vi "Clear_TemporaryFiles.vi"() -> ()   [LabVIEW 2018]
panel:
  out "text":string
  in  "EventCodes_U64Arr in":u64[](array[numeric])
  out "data":u64[](array[numeric])
  out "All Files in Dir":path[](array[path])
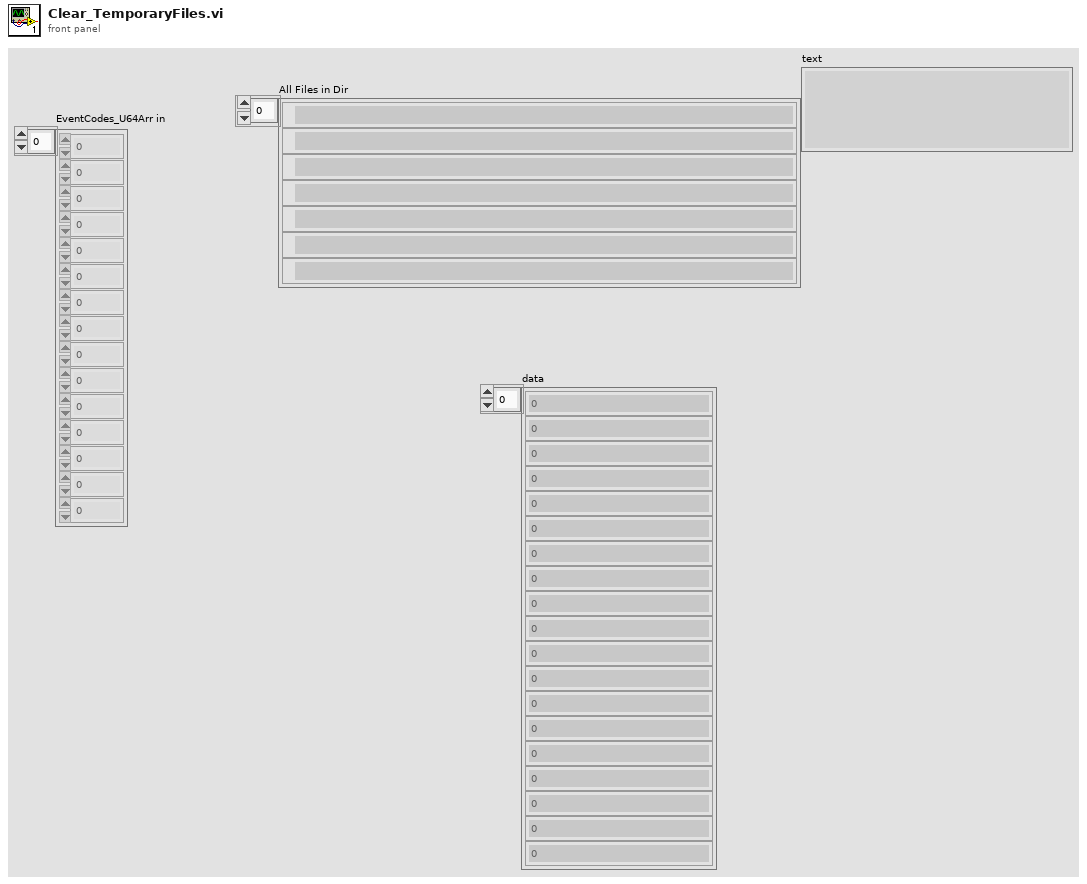
[diagram p1: front panel]
types:
  T1 = enum16{"open", "replace", "create", "open or create", "replace or create", "replace or create with confirmation"}
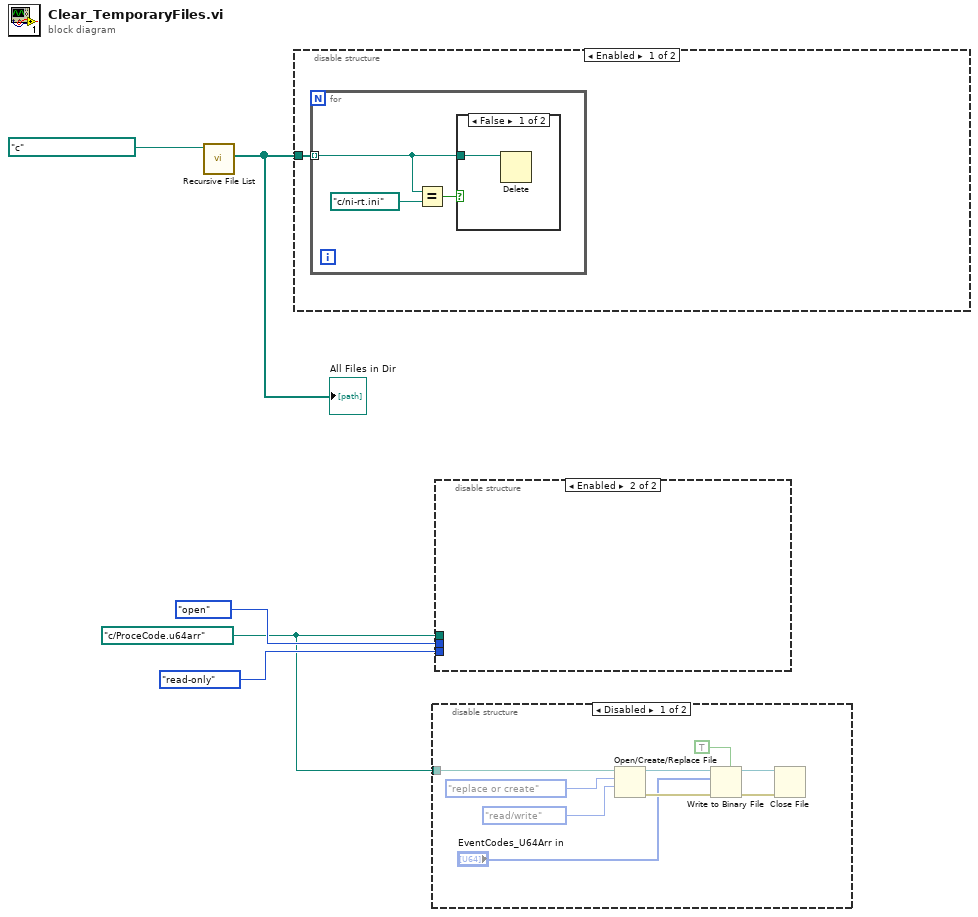
[diagram p0: block diagram]
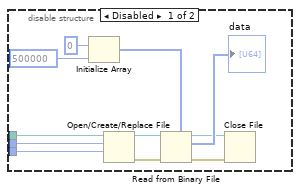
[diagram p3: hidden frame]
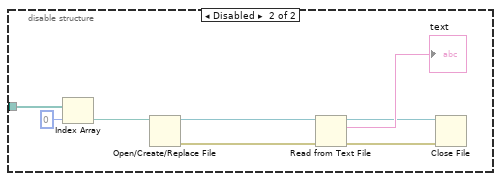
[diagram p5: hidden frame]
diagram:
  w2 = path "c:/ProceCode.u64arr" ("file path (use dialog)")
  n1 = call <vilib>:"Recursive File List.vi"("Folder Path"=path "c:/" ("file path (use dialog)")) -> ("All Files in Dir"=w1:path[])  [unwired: 6 in, 4 out]
  "All Files in Dir" <- w1
  n2 = disable-structure shown="Enabled" {
    disable-tunnel: w1 -> [w6 w18]
    frame Enabled {
      n3 = for {
        tunnel: w6 -> [w7] mode=indexing
        n4 = Equal?(x=w7, y=path "c:/ni-rt.ini") -> (x = y?=w8:bool)
        n5 = case shown="False" w8 {
          tunnel: w7 -> [w10 _]
          frame False {
            n6 = Delete(path (use dialog)=w10) -> ()  [unwired: 4 in, 3 out]
          }
          frame True {
          }
        }
      }
    }
    frame Disabled {
      n7 = Index Array(array=w18, index=0) -> (element=w16:path)
      n8 = Open/Create/Replace File(file path (use dialog)=w16) -> (refnum out=w15:refnum<file>, error out=w14:errorcluster)  [unwired: 5 in, 1 out]
      n9 = Read from Text File(file (use dialog)=w15, error in=w14) -> (refnum out=w12:refnum<file>, text=→"text":string, error out=w11:errorcluster)  [unwired: 2 in, 1 out]
      n10 = Close File(refnum=w12, error in=w11) -> ()  [unwired: 2 out]
    }
  }
  n11 = disable-structure shown="Disabled" {
    disable-tunnel: w2 -> [w20 _]
    frame Disabled {
      n12 = Open/Create/Replace File(file path (use dialog)=w20, operation (0:open)=T1."replace or create", access (0:read/write)=enum16{"read/write", "read-only", "write-only"}."read/write") -> (refnum out=w26:refnum<file>, error out=w25:errorcluster)  [unwired: 3 in, 1 out]
      n13 = Write to Binary File(file (use dialog)=w26, data="EventCodes_U64Arr in", error in=w25, 5:TRUE ("prepend array or string size? (T)")) -> (refnum out=w23:refnum<file>, error out=w22:errorcluster)  [unwired: 2 in, 1 out]
      n14 = Close File(refnum=w23, error in=w22) -> ()  [unwired: 2 out]
    }
    frame Enabled {
    }
  }
  n15 = disable-structure shown="Enabled" {
    disable-tunnel: T1."open" ("operation (0:open)") -> [w36 _]
    disable-tunnel: enum16{"read/write", "read-only", "write-only"}."read-only" ("access (0:read/write)") -> [w35 _]
    disable-tunnel: w2 -> [w28 _]
    frame Disabled {
      n16 = Initialize Array(u64 0, 500000 ("dimension size")) -> (w32:u64[])
      n17 = Open/Create/Replace File(file path (use dialog)=w28, operation (0:open)=w36, access (0:read/write)=w35) -> (refnum out=w37:refnum<file>, error out=w29:errorcluster)  [unwired: 3 in, 1 out]
      n18 = Read from Binary File(5:w32, 8:w29, 11:w37) -> (0:w38:errorcluster, 2:→"data":u64[], 3:w30:refnum<file>)  [unwired: 3 in, 1 out]
      n19 = Close File(refnum=w30, error in=w38) -> ()  [unwired: 2 out]
    }
    frame Enabled {
    }
  }
